vi "LSX Get BPZ Trackball Factor.vi"(8 "error in (no error)":errorcluster, 10 "pdAValue":dbl, 11 "lLSID":i32) -> (0 "error out":errorcluster, 2 "pdAValue out":dbl, 3 "function return":i32)   [LabVIEW 2016, in "Tango_DLL.lvlib"]
doc: "TANGOAPI int TANGOCALL LSX_GetBPZTrackballFactor (int lLSID, double *pdAValue);"
uses:
  Tango_DLL.lvlib
  2017/Microscope Control/Device Library/Stages/Marzhauser/SCAN IM 120 x 80/Tango DLL VIs/Tango_DLL.dll
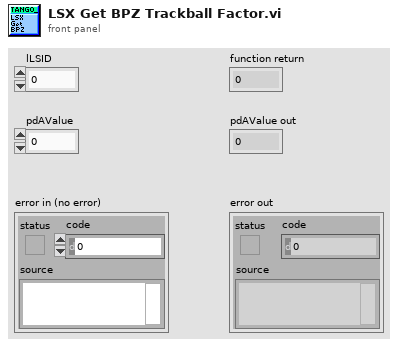
[diagram p1: front panel]
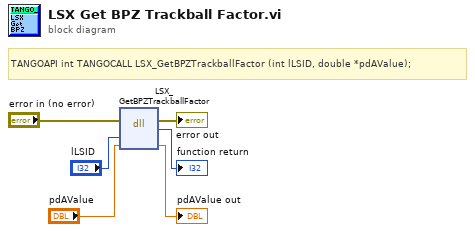
[diagram p0: block diagram]
diagram:
  # "TANGOAPI int TANGOCALL LSX_GetBPZTrackballFactor (int lLSID, double *pdAValue);"
  n1 = dll-call lib="C:/Users/4PiSMS/Documents/Microscope Control/2017/Microscope Control/Device Library/Stages/Marzhauser/SCAN IM 120 x 80/Tango DLL VIs/Tango_DLL.*" fn="LSX_GetBPZTrackballFactor"(error in="error in (no error)", "lLSID"="lLSID", "pdAValue"="pdAValue") -> (error out=→"error out":errorcluster, →"function return":i32, "pdAValue"=→"pdAValue out":dbl)  [unwired: 3 in, 1 out]
